vi "Read String Format.vi"(8 "error in (no error)":errorcluster, 11 "String Log Sink in":refnum<class "String Log Sink.lvclass">) -> (0 "error out":errorcluster, 2 "String Format":refnum<class "IStringFormat.lvclass">, 3 "String Log Sink out":refnum<class "String Log Sink.lvclass">)   [LabVIEW 2019, in "String Log Sink.lvclass"]
uses:
  <vilib>/gpm_packages/@cs/event-logger/Source/String Log Sink/String Log Sink.lvclass
  <vilib>/gpm_packages/@cs/event-logger/Source/IStringFormat/IStringFormat.lvclass
  <vilib>/gpm_packages/@cs/event-logger/Source/String Log Sink/String Log Sink.lvclass/String Log Sink.ctl
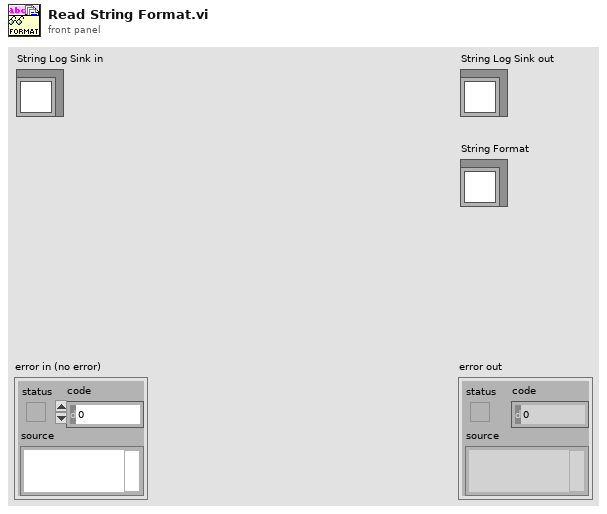
[diagram p1: front panel]
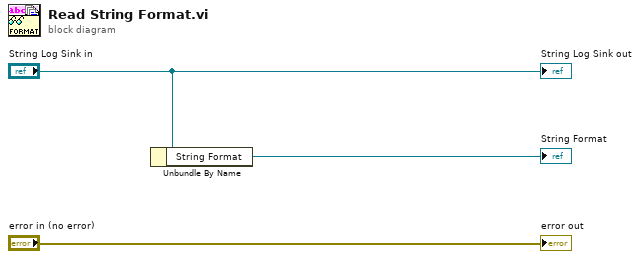
[diagram p0: block diagram]
diagram:
  n1 = Unbundle By Name("String Log Sink in") -> ("String Format"=→"String Format":refnum<class "IStringFormat.lvclass">)
  "error out" <- "error in (no error)"
  "String Log Sink out" <- "String Log Sink in"
